vi "Errors.vi"   [LabVIEW 2017, in "DSF Core.lvlib" / "ID Pool.lvclass"]
uses:
  ID Pool.lvclass
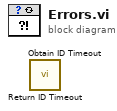
[diagram p0: block diagram]
diagram:
  n1 = call "Return ID Timeout.vi"() -> ()  [unwired: 10 in, 2 out]
  n2 = call "Obtain ID Timeout.vi"() -> ()  [unwired: 10 in, 2 out]
